vi "test_Path (programdata).vi"(8 "error in (no error)":errorcluster, 11 "TestCase in":refnum<class "Read Section - Path Tests.lvclass">) -> (0 "error out":errorcluster, 3 "TestCase out":refnum<class "Read Section - Path Tests.lvclass">)   [LabVIEW 2017, in "Read Section - Path Tests.lvclass"]
uses:
  Read Section - Path Tests.lvclass
  C:/Development/Reuse-libraries/File IO/_Unit Test/Read File Tests/Read File Tests.lvclass
  Read File Tests.lvclass/Read File Tests.ctl
  Read/Read Section - Path.vi
  <vilib>/addons/_JKI Toolkits/VI Tester/TestCase.llb/TestCase.lvclass
  TSC File IO.lvlib
  Read File Tests.lvclass
  C:/Program Files (x86)/National Instruments/LabVIEW 2017/vi.lib/addons/_JKI Toolkits/VI Tester/TestCase.llb/TestCase.lvclass
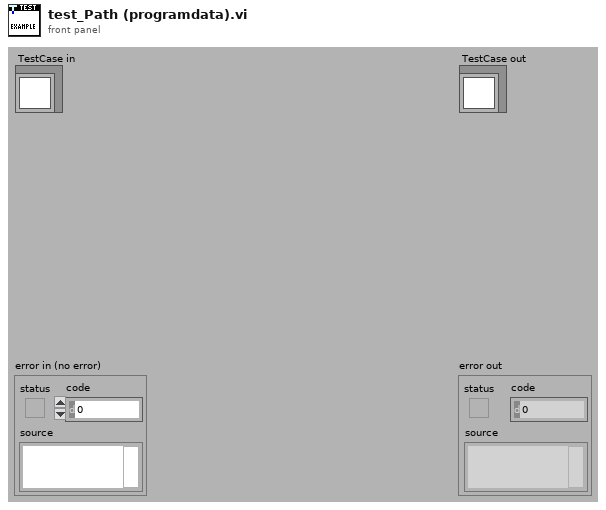
[diagram p1: front panel]
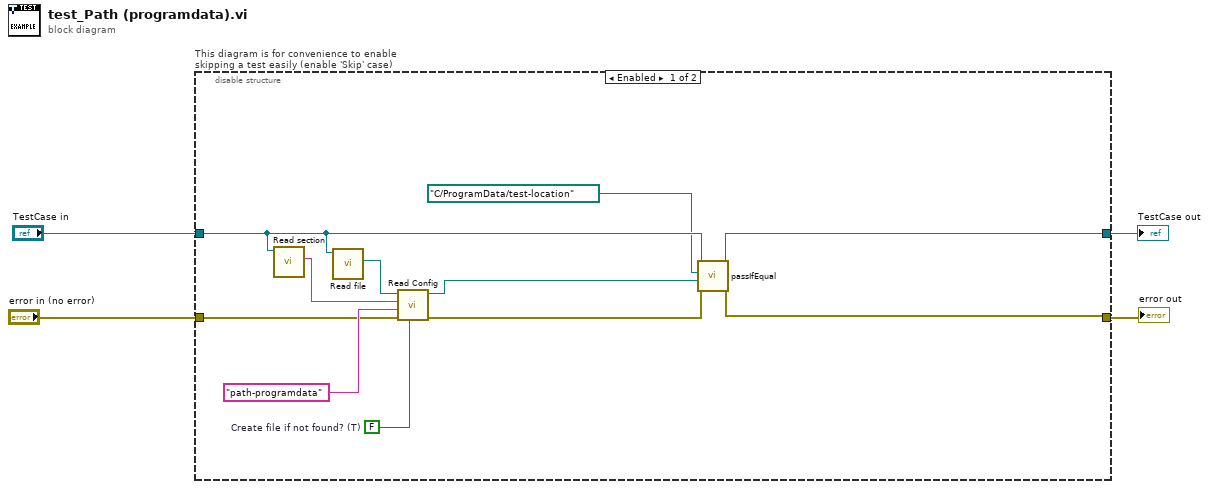
[diagram p0: block diagram]
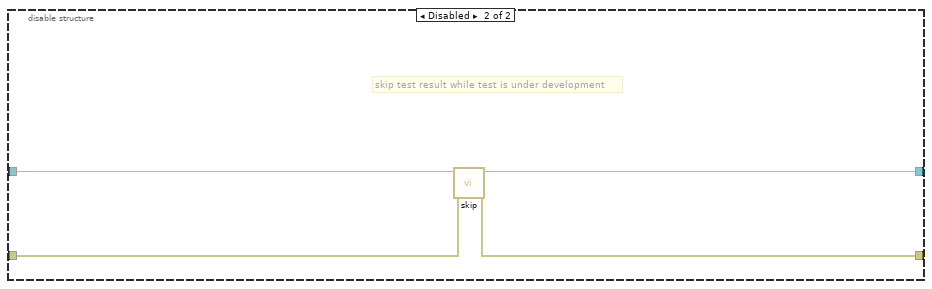
[diagram p2: hidden frame]
diagram:
  n1 = disable-structure "This diagram is for convenience to enable skipping a test easily (enable 'Skip' case)" shown="Enabled" {
    disable-tunnel: "TestCase in" -> [w8 w19]
    disable-tunnel: [w15 w17] -> w1
    disable-tunnel: [w14 w18] -> w3
    disable-tunnel: "error in (no error)" -> [w11 w16]
    frame Enabled {
      w12 = FALSE  # Create file if not found? (T)
      n2 = call "Read section.vi"("Read File Tests in"=w8) -> ("section"=w7:string)  [unwired: 8 in, 2 out]
      n3 = call "Read file.vi"("Read File Tests in"=w8) -> ("file"=w9:path)  [unwired: 8 in, 2 out]
      n4 = call-poly "Read Config.vi"("Create file if not found? (T)"=w12, "error in (no error)"=w11, "key"="path-programdata", "section"=w7, "Path"=w9) -> ("error out"=w10:errorcluster, "value"=w6:path)  [unwired: 5 in]
      n5 = call-dynamic "passIfEqual.vi"("error in (no error)"=w10, "y"=w6, "x"=path "C:/ProgramData/test-location", "TestCase in"=w8) -> ("error out"=w14:errorcluster, "TestCase out"=w15:refnum<class "Read Section - Path Tests.lvclass">)  [unwired: 6 in]
    }
    frame Disabled {
      # "skip test result while test is under development"
      n6 = call <vilib>:"skip.vi"("error in (no error)"=w16, "TestCase in"=w19) -> ("error out"=w18:errorcluster, "TestCase out"=w17:refnum<class "Read Section - Path Tests.lvclass">)  [unwired: 8 in]
    }
  }
  "error out" <- w3
  "TestCase out" <- w1
